vi "39.vi"() -> ()   [LabVIEW 2021]
uses:
  2b6e569c-fb92-48e0-adc9-2269a59834e4.vi
  <vilib>/Comparison/Less/Less Functor/Less Functor.lvclass
panel:
  in  "p_max":i32=1000
  out "reversed array":T1(array[cluster])
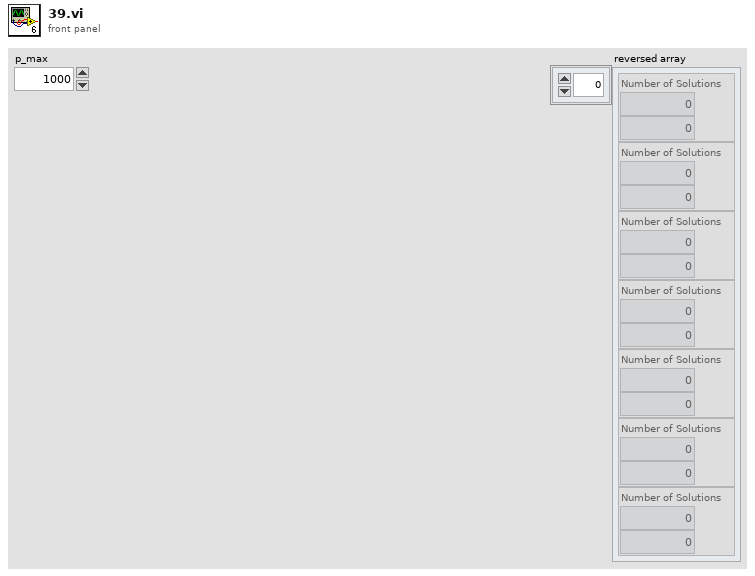
[diagram p1: front panel]
types:
  T1 = cluster{"Number of Solutions":i32, "Numeric":i32}[]
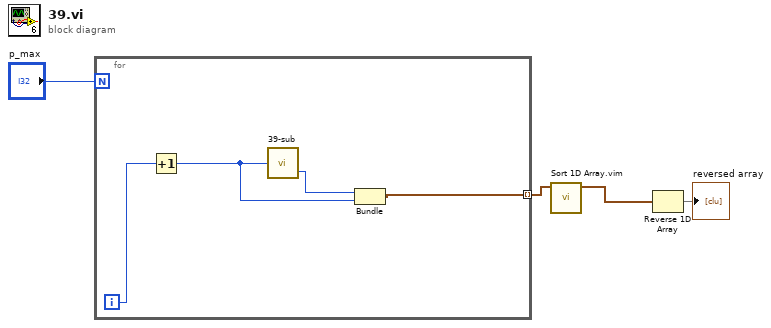
[diagram p0: block diagram]
diagram:
  n1 = for {
    N: "p_max" -> [_]
    tunnel: [w5] -> w3 mode=indexing
    i -> [w8]
    n2 = Increment(x=w8) -> (x+1=w6:i32)
    n3 = call "39-sub.vi"("p"=w6) -> ("Number of Solutions"=w7:i32)  [unwired: 1 out]
    n4 = Bundle("Number of Solutions"=w7, w6) -> (w5:cluster{"Number of Solutions":i32, i32})  [unwired: 1 in]
  }
  n5 = call "Sort 1D Array.vim"("unsorted array"=w3) -> ("sorted array"=w2:cluster{"Number of Solutions":i32, i32}[])  [unwired: 10 in]
  n6 = Reverse 1D Array(array=w2) -> (reversed array=→"reversed array":cluster{"Number of Solutions":i32, i32}[])
